vi "TestACQ.vi"() -> ()   [LabVIEW 2014]
uses:
  <vilib>/DAQmx/configure/trigger.llb/DAQmx Start Trigger (Digital Edge).vi
  <vilib>/DAQmx/configure/timing.llb/DAQmx Timing (Implicit).vi
  <vilib>/DAQmx/configure/timing.llb/DAQmx Timing (Sample Clock).vi
  <vilib>/DAQmx/read.llb/DAQmx Read (Analog 2D I16 NChan NSamp).vi
  <vilib>/DAQmx/write.llb/DAQmx Write (Analog 1D DBL NChan 1Samp).vi
  <vilib>/DAQmx/write.llb/DAQmx Write (Digital 1D Bool NChan 1Samp 1Line).vi
  <vilib>/DAQmx/write.llb/DAQmx Write (Digital Bool 1Line 1Point).vi
  <resource>/objmgr/daqmx.rc
panel:
  out "size(s) 2":i32
  in  "Red":bool
  out "error out 4":errorcluster
  in  "Power":bool[](array[boolean])=[FALSE, FALSE, FALSE, FALSE, FALSE]
  out "number of samples written per channel 3":u32
  out "number of samples written per channel 2":u32
  in  "PMT":dbl[](array[numeric])=[4.0, 4.0, 4.0, 4.0, 4.0] format="%0.2f"
  in  "Laser Power":dbl[](array[numeric])=[3.0, 3.0, 3.0] format="%0.2f"
  out "number of samples written per channel":u32
  in  "Enable":bool[](array[boolean])=[FALSE, FALSE]
  out "Waveform Graph":i64[][](graph)
  out "size(s)":i32[](array[numeric])
  out "error out 2":errorcluster
  in  "Stop Button":bool
  out "error out":errorcluster
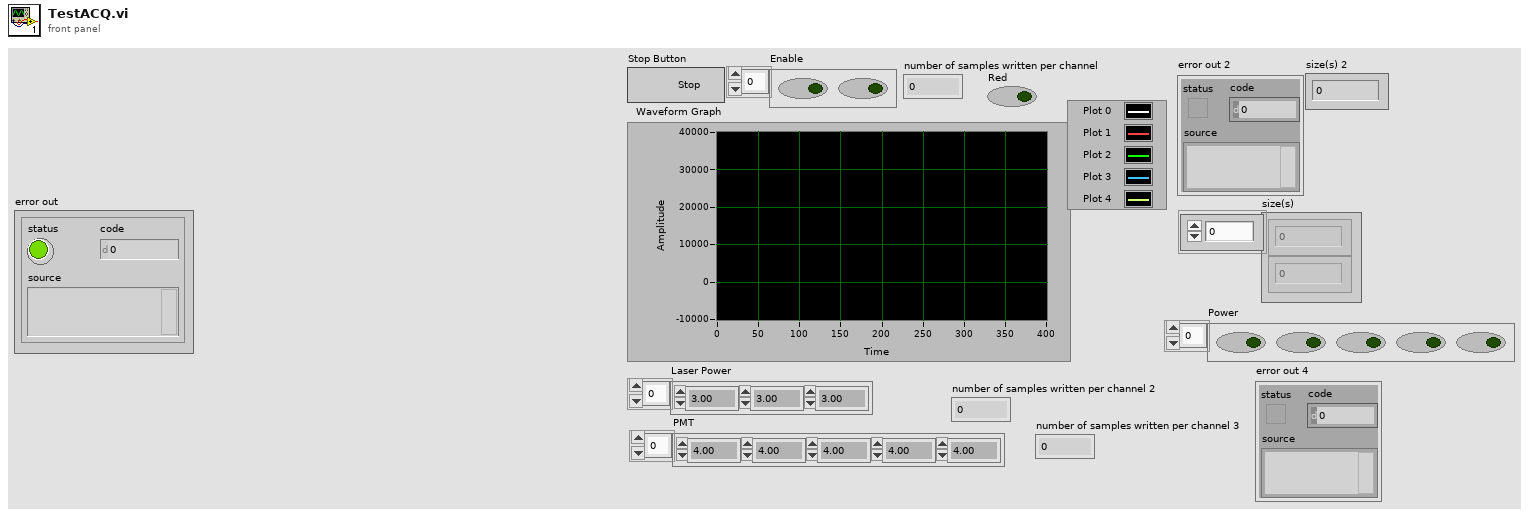
[diagram p1: front panel]
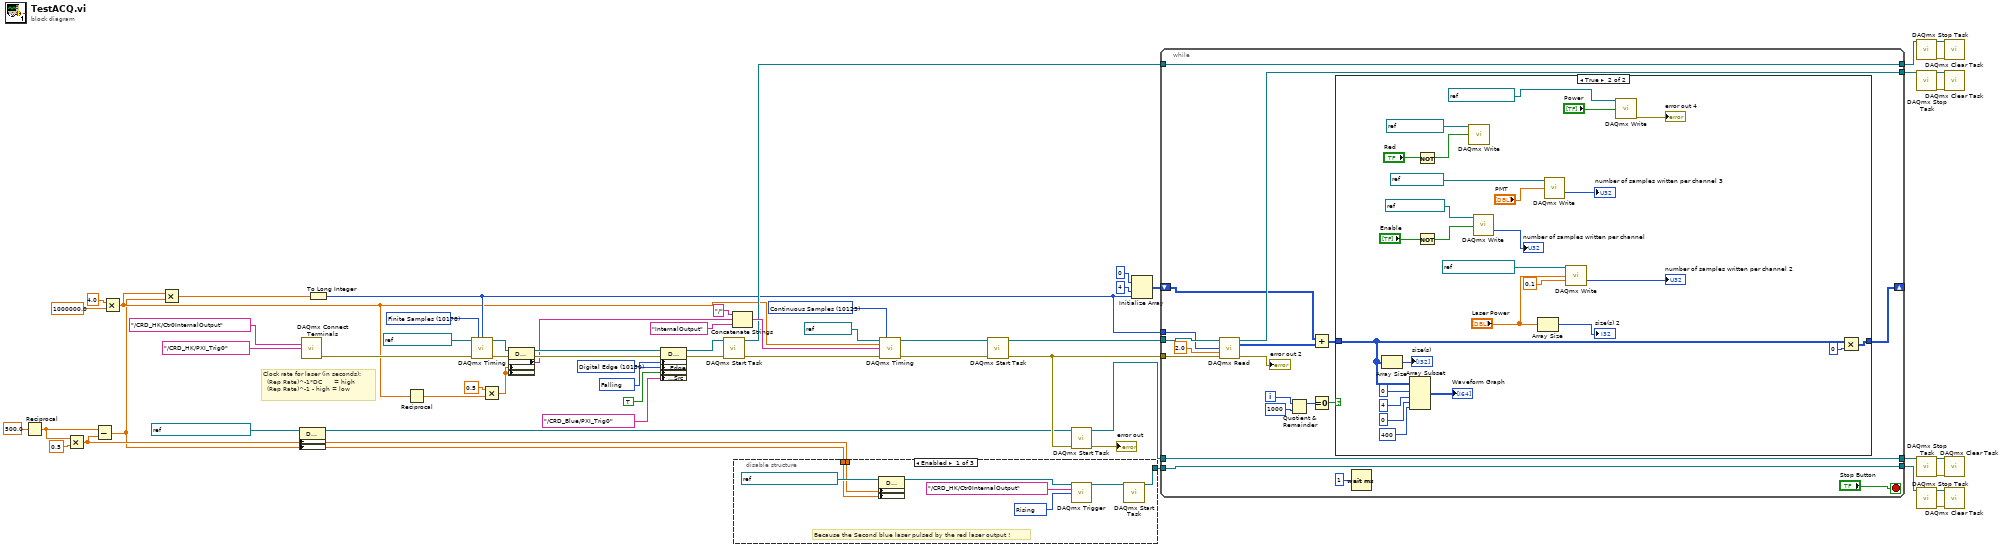
[diagram p0: block diagram]
diagram:
  w60 = 10123 items=["Finite Samples"=10178, "Continuous Samples"=10123, "Hardware Timed Single Point"=12522] ("sample mode")
  w48 = 10171 items=["Rising"=10280, "Falling"=10171] ("Ref.DigEdge.Edge")
  w47 = 10150 items=["Analog Edge"=10099, "Digital Edge"=10150, "Digital Pattern"=10398, "Analog Window"=10103, "None"=10230] ("Ref.TrigType")
  w40 = 10178 items=["Finite Samples"=10178, "Continuous Samples"=10123, "Hardware Timed Single Point"=12522] ("sample mode")
  # "Clock rate for laser (in seconds):\n  (Rep Rate)^-1*DC      = high\n  (Rep Rate)^-1 - high = low"
  n1 = Reciprocal(x=500.0) -> (1/x=w35:dbl)
  n2 = Multiply(x=w35, y=0.5) -> (x*y=w6:dbl)
  n3 = Subtract(x=w35, y=w6) -> (x-y=w5:dbl)
  n4 = Multiply(x=4.0, y=1000000.0) -> (x*y=w9:dbl)
  n5 = Multiply(x=w9, y=w5) -> (x*y=w34:dbl)
  n6 = property class="DAQmx Channel"(reference=refnum<k21> "CRDS laser pulse" ("DO"), "CO.Pulse.HighTime"=w6, "CO.Pulse.LowTime"=w5) -> (reference out=w7:refnum<k21>)  [unwired: 1 in, 1 out]
  n7 = call <vilib>:"DAQmx Connect Terminals.vi"("source terminal"=tag "/CRD_HK/Ctr0InternalOutput", "destination terminal"=tag "/CRD_HK/PXI_Trig0") -> ("error out"=w57:errorcluster)  [unwired: 13 in]
  n8 = To Long Integer(number=w34) -> (32bit integer=w10:i32)
  n9 = Reciprocal(x=w9) -> (1/x=w37:dbl)
  n10 = call-poly <vilib>:"DAQmx Timing.vi"("task/channels in"=refnum<k21> "CRDS clock", "sample mode"=w40, "samples per channel"=w10, "error in"=w57) -> ("task out"=w41:refnum<k21>, "error out"=w50:errorcluster)  [unwired: 10 in]
  n11 = Multiply(x=0.5, y=w37) -> (x*y=w11:dbl)
  n12 = property class="DAQmx Channel"(reference=w41, error in=w50, "CO.Pulse.HighTime"=w11, "CO.Pulse.LowTime"=w11) -> (reference out=w46:refnum<k21>, error out=w51:errorcluster, "PhysicalChanName"=w44:tag)
  n13 = property class="DAQmx Trigger"(reference=w46, error in=w51, "Start.TrigType"=w47, "Start.DigEdge.Edge"=w48, "Start.Retriggerable"=TRUE, "Start.DigEdge.Src"=tag "/CRD_Blue/PXI_Trig0") -> (reference out=w52:refnum<k21>, error out=w53:errorcluster)
  n14 = call <vilib>:"DAQmx Start Task.vi"("task/channels in"=w52, "error in"=w53) -> ("task out"=w26:refnum<k21>, "error out"=w39:errorcluster)  [unwired: 12 in]
  n15 = Concatenate Strings("/" ("string"), w44, "InternalOutput" ("string")) -> (w45:string)
  n16 = disable-structure shown="Enabled" {
    disable-tunnel: w6 -> [w63 _ _]
    disable-tunnel: w5 -> [w62 _ _]
    disable-tunnel: [w61 _ _] -> w4
    frame Enabled {
      w65 = 10280 items=["Rising"=10280, "Falling"=10171] ("edge")
      # "Because the Second blue laser pulsed by the red laser output !"
      n17 = property class="DAQmx Channel"(reference=refnum<k21> "CRD Red Laser Output" ("task"), "CO.Pulse.HighTime"=w63, "CO.Pulse.LowTime"=w62) -> (reference out=w67:refnum<k21>)  [unwired: 1 in, 1 out]
      n18 = call-poly <vilib>:"DAQmx Trigger.vi"("task/channels in"=w67, "source"=tag "/CRD_HK/Ctr0InternalOutput" ("source terminal"), "edge"=w65) -> ("task out"=w64:refnum<k21>)  [unwired: 11 in, 1 out]
      n19 = call <vilib>:"DAQmx Start Task.vi"("task/channels in"=w64) -> ("task out"=w61:refnum<k21>)  [unwired: 13 in, 1 out]
    }
    frame Disabled {
    }
    frame Disabled {
    }
  }
  n20 = call-poly <vilib>:"DAQmx Timing.vi"("task/channels in"=refnum<k21> "CRDS AI", "sample mode"=w60, "rate"=w9, "source"=w45, "error in"=w39) -> ("task out"=w54:refnum<k21>, "error out"=w55:errorcluster)  [unwired: 9 in]
  n21 = call <vilib>:"DAQmx Start Task.vi"("task/channels in"=w54, "error in"=w55) -> ("task out"=w28:refnum<k21>, "error out"=w8:errorcluster)  [unwired: 12 in]
  n22 = call <vilib>:"DAQmx Start Task.vi"("task/channels in"=w7, "error in"=w8) -> ("task out"=w27:refnum<k21>, "error out"=→"error out":errorcluster)  [unwired: 12 in]
  n23 = Initialize Array(i64 0, 4 ("dimension size"), w10) -> (w12:i64[][])
  n24 = while {
    tunnel: w28 -> [w87]
    tunnel: [w86] -> w23
    tunnel: w27 -> [w85]
    tunnel: [w85] -> w25
    tunnel: w26 -> [w84]
    tunnel: [w84] -> w24
    tunnel: w10 -> [w81]
    tunnel: w8 -> [w76]
    shift-right: [w70] -> _
    shift-left: w12 -> [w73]
    tunnel: w4 -> [w69]
    tunnel: [w69] -> w3
    i -> [w80]
    stop <- "Stop Button" stop-if-true
    n25 = call-poly <vilib>:"DAQmx Read.vi"("task/channels in"=w87, "number of samples per channel"=w81, "timeout"=2.0, "error in"=w76) -> ("task out"=w86:refnum<k21>, "data"=w72:i16[][], "error out"=→"error out 2":errorcluster)  [unwired: 9 in]
    n26 = Quotient & Remainder(x=w80, y=1000) -> (x-y*floor(x/y)=w79:i32)  [unwired: 1 out]
    n27 = Add(x=w73, y=w72) -> (x+y=w71:i64[][])
    n28 = Equal To 0?(x=w79) -> (x = 0?=w78:bool)
    n29 = case shown="True" w78 {
      tunnel: w71 -> [w88 w99]
      tunnel: [w88 w97] -> w70
      frame False {
      }
      frame True {
        n30 = Array Size(array=w99) -> (size(s)=→"size(s)":i32[])
        n31 = Array Subset(array=w99, index (row)=0 ("index"), length (row)=4 ("length"), index (col)=0 ("index"), length (col)=400 ("length")) -> (→"Waveform Graph":i64[][])
        n32 = Not(x="Red") -> (.not. x?=w100:bool)
        n33 = Not(x="Enable") -> (.not. x?=w101:bool[])
        n34 = call-poly <vilib>:"DAQmx Write.vi"("task/channels in"=refnum<k21> "Red Enable", "data"=w100) -> ()  [unwired: 11 in, 3 out]
        n35 = call-poly <vilib>:"DAQmx Write.vi"("task/channels in"=refnum<k21> "Blue Enable", "data"=w101) -> ("number of samples written per channel"=→"number of samples written per channel":u32)  [unwired: 11 in, 2 out]
        n36 = Array Size(array="Laser Power") -> (size(s)=→"size(s) 2":i32)
        n37 = call-poly <vilib>:"DAQmx Write.vi"("task/channels in"=refnum<k21> "PMT Gain", "data"="PMT") -> ("number of samples written per channel"=→"number of samples written per channel 3":u32)  [unwired: 11 in, 2 out]
        n38 = call-poly <vilib>:"DAQmx Write.vi"("task/channels in"=refnum<k21> "CRD Laser Gain", "data"="Laser Power", "timeout"=0.1) -> ("number of samples written per channel"=→"number of samples written per channel 2":u32)  [unwired: 10 in, 2 out]
        n39 = call-poly <vilib>:"DAQmx Write.vi"("task/channels in"=refnum<k21> "Power Supply", "data"="Power") -> ("error out"=→"error out 4":errorcluster)  [unwired: 11 in, 2 out]
        n40 = Multiply(x=w99, y=i16 0) -> (x*y=w97:i64[][])
      }
    }
    n41 = Wait (ms)(milliseconds to wait=u32 1) -> ()  [unwired: 1 out]
  }
  n42 = call <vilib>:"DAQmx Stop Task.vi"("task/channels in"=w24) -> ("task out"=w18:refnum<k21>, "error out"=w17:errorcluster)  [unwired: 13 in]
  n43 = call <vilib>:"DAQmx Stop Task.vi"("task/channels in"=w23) -> ("task out"=w20:refnum<k21>, "error out"=w19:errorcluster)  [unwired: 13 in]
  n44 = call <vilib>:"DAQmx Stop Task.vi"("task/channels in"=w25) -> ("task out"=w16:refnum<k21>, "error out"=w15:errorcluster)  [unwired: 13 in]
  n45 = call <vilib>:"DAQmx Stop Task.vi"("task/channels in"=w3) -> ("task out"=w2:refnum<k21>, "error out"=w1:errorcluster)  [unwired: 13 in]
  n46 = call <vilib>:"DAQmx Clear Task.vi"("task in"=w18, "error in"=w17) -> ()  [unwired: 13 in, 1 out]
  n47 = call <vilib>:"DAQmx Clear Task.vi"("task in"=w20, "error in"=w19) -> ()  [unwired: 13 in, 1 out]
  n48 = call <vilib>:"DAQmx Clear Task.vi"("task in"=w16, "error in"=w15) -> ()  [unwired: 13 in, 1 out]
  n49 = call <vilib>:"DAQmx Clear Task.vi"("task in"=w2, "error in"=w1) -> ()  [unwired: 13 in, 1 out]
